vi "Main Engine Send Hardware Info.vi"(5 "Q Cluster":T6, 6 "Hardware Info":T1[](array[typedef]) {"Is Present?" items=["Initializing"=-2, "Unknown"=-1, "Not Present"=0, "Present"=1]}, 7 "DAQ Device Info":T8[](array[typedef]), 8 "error in":errorcluster, 9 "Ethernet IP Address":string[](array[string]), 10 "Serial Device Info":T7[](array[typedef])) -> (0 "error out":errorcluster)   [LabVIEW 2021]
doc: "All Rights Reserved © 2023 SyncSols"
uses:
  Controls/Main Engine DAQ Device Info.ctl
  Controls/Main Engine Serial Card Details.ctl
  Controls/Main Engine Q Cluster.ctl
  Controls/RT HW Info.ctl
  Controls/Main Engine Serial Info JSON Data.ctl
  Controls/Main Engine DAQ Harware Info JSON Data.ctl
  Controls/Main Engine Ehernet IP Address JSON Data.ctl
  Controls/Main Engine Hardware Info Data Cluster.ctl
  Host-Control's/TCP Tx-Rx cluster.ctl
  <vilib>/addons/_JKI.lib/Serialization/JSON/JKI JSON Serialization.lvlib
panel:
  in  "output cluster":T2
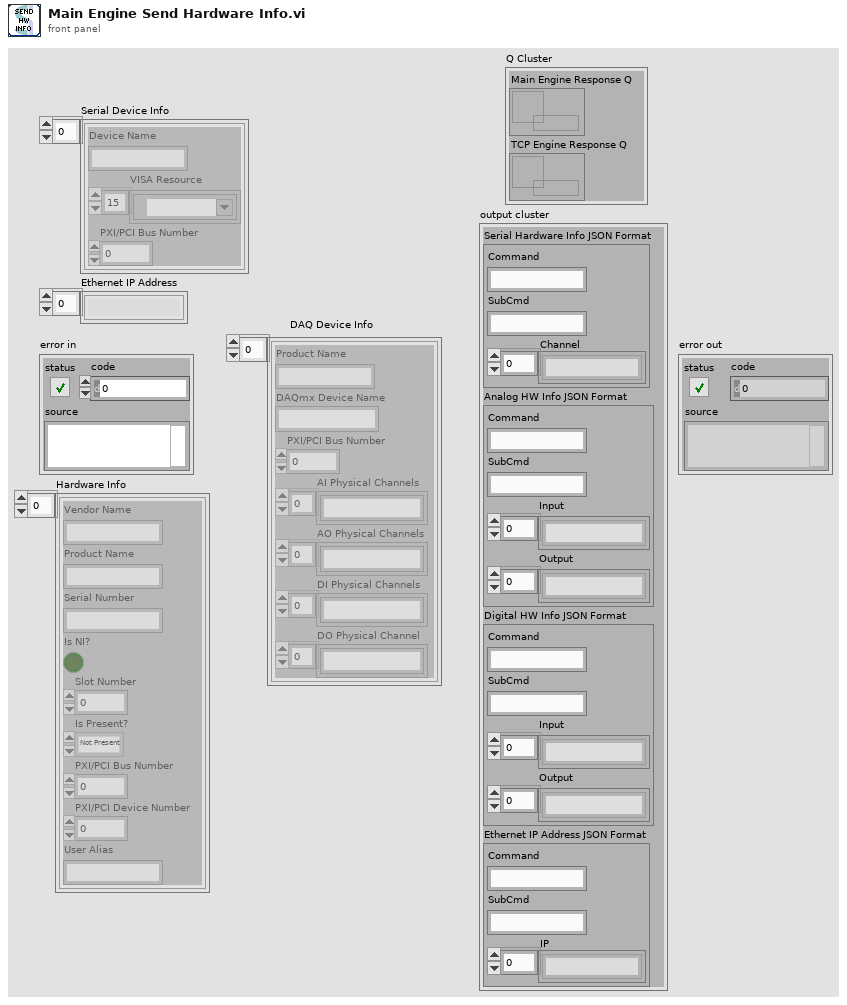
[diagram p1: front panel]
types:
  T1 = typedef "Main Engine Hardware Info Data Cluster.ctl" = cluster{"Vendor Name":string, "Product Name":string, "Serial Number":string, "Is NI?":bool, "Slot Number":i32, "Is Present?":i32, "PXI/PCI Bus Number":u32, "PXI/PCI Device Number":u32, "User Alias":string}
  T2 = typedef "RT HW Info.ctl" = cluster{"Serial Hardware Info JSON Format":T3, "Analog HW Info JSON Format":T4, "Digital HW Info JSON Format":T4, "Ethernet IP Address JSON Format":T5}
  T3 = typedef "Main Engine Serial Info JSON Data.ctl" = cluster{"Command":string, "SubCmd":string, "Channel":string[]}
  T4 = typedef "Main Engine DAQ Harware Info JSON Data.ctl" = cluster{"Command":string, "SubCmd":string, "Input":string[], "Output":string[]}
  T5 = typedef "Main Engine Ehernet IP Address JSON Data.ctl" = cluster{"Command":string, "SubCmd":string, "IP":string[]}
  T6 = typedef "Main Engine Q Cluster.ctl" = cluster{"Main Engine Response Q":refnum<queue>, "TCP Engine Response Q":refnum<queue>}
  T7 = typedef "Main Engine Serial Card Details.ctl" = cluster{"Device Name":string, "VISA Resource":refnum<visa-resource-name>[], "PXI/PCI Bus Number":u32}
  T8 = typedef "Main Engine DAQ Device Info.ctl" = cluster{"Product Name":string, "DAQmx Device Name":string, "PXI/PCI Bus Number":u32, "AI Physical Channels":string[], "AO Physical Channels":string[], "DI Physical Channels":string[], "DO Physical Channel":string[]}
  T9 = typedef "TCP Tx-Rx cluster.ctl" = cluster{"Interface":string, "Command":string, "SubCmd":string, "Data":variant}
  T10 = cluster{"DAQ Device Info":T8[], "Ethernet IP Address":string[]}
  T11 = cluster{"Serial Hardware Info JSON Format":T3, "Analog HW Info JSON Format":T4, "Digital HW Info JSON Format":T4, "Ethernet IP Address JSON Format":T5}
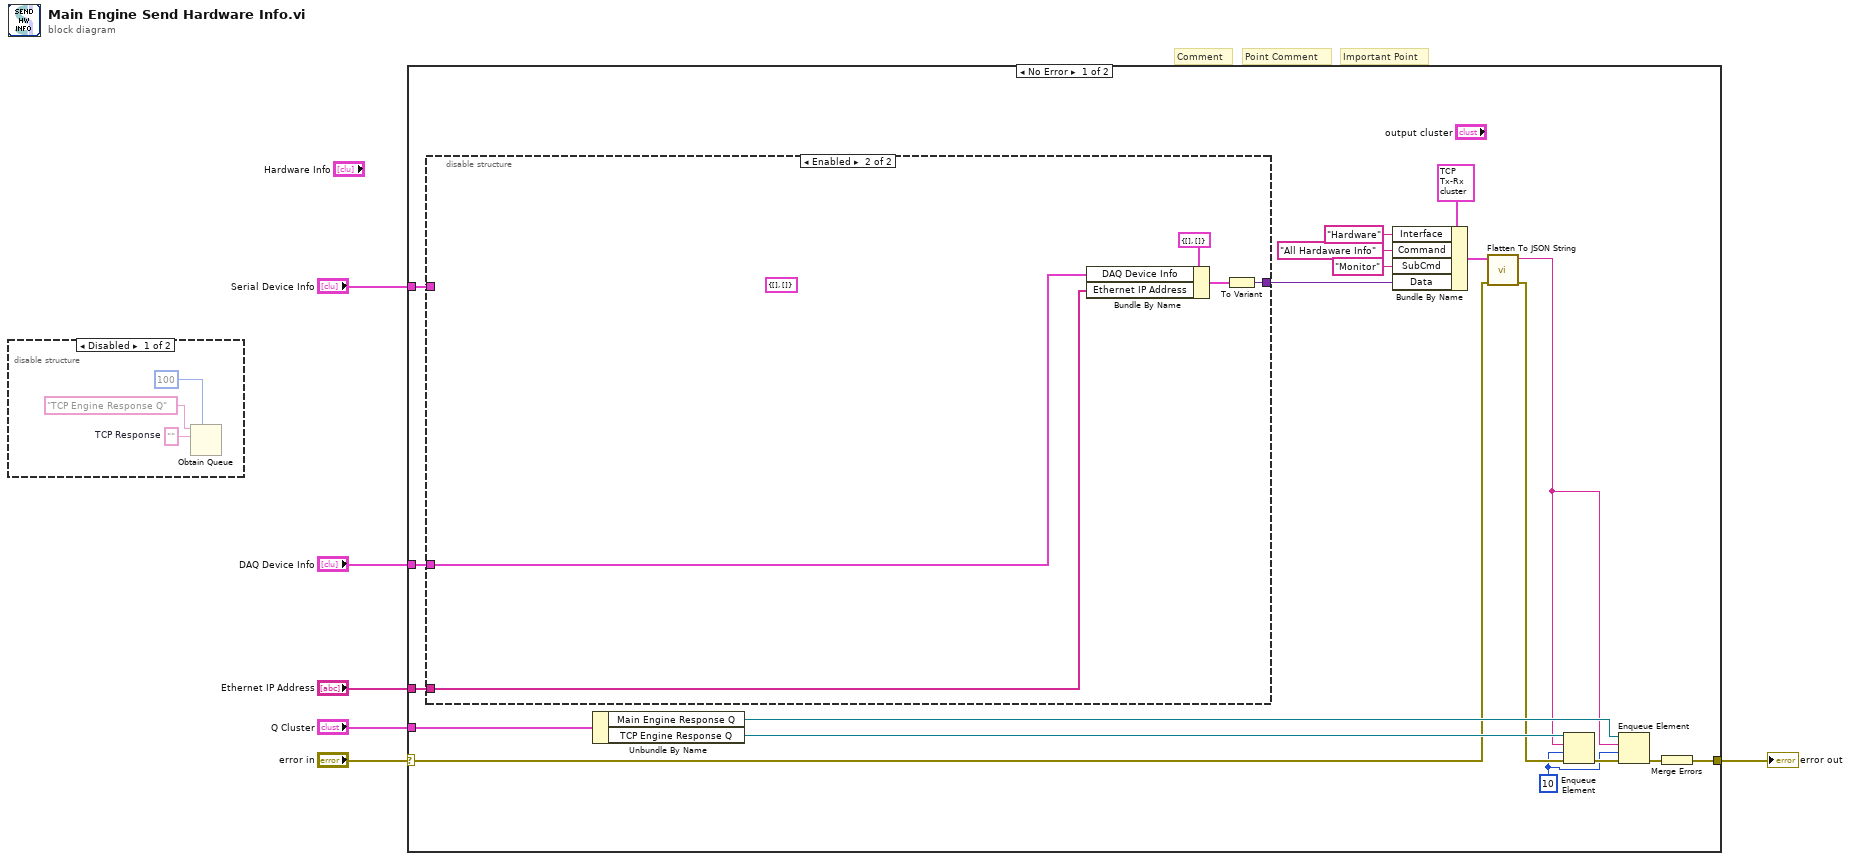
[diagram p0: block diagram]
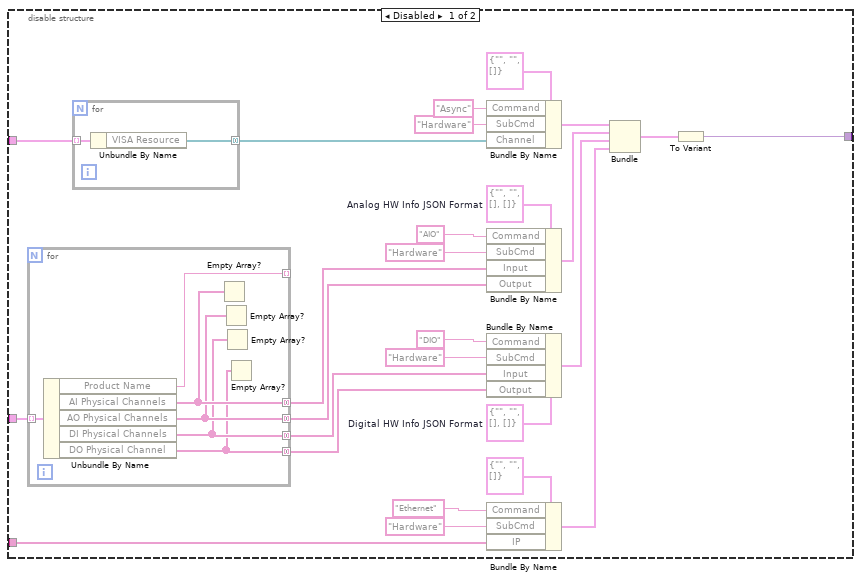
[diagram p3: hidden frame]
diagram:
  # "Important Point"
  # "Point Comment"
  # "Comment"
  n1 = disable-structure shown="Disabled" {
    frame Disabled {
      w9 = ""  # TCP Response
      n2 = Obtain Queue(max queue size (-1, unlimited)=100, name (unnamed)="TCP Engine Response Q", element data type=w9) -> ()  [unwired: 2 in, 3 out]
    }
    frame Enabled {
    }
  }
  n3 = case shown="No Error" "error in" {
    selector: "error in" -> [w13 w68]
    tunnel: [w25 w68] -> w6
    tunnel: "DAQ Device Info" -> [w28 _]
    tunnel: "Serial Device Info" -> [w27 _]
    tunnel: "Ethernet IP Address" -> [w23 _]
    tunnel: "Q Cluster" -> [w22 _]
    frame No Error {
      w10 = 10 ("timeout in ms (-1)")
      n4 = disable-structure shown="Enabled" {
        disable-tunnel: w28 -> [w54 w63]
        disable-tunnel: w27 -> [w48 _]
        disable-tunnel: w23 -> [w36 w66]
        disable-tunnel: [w29 w67] -> w16
        frame Disabled {
          w51 = T4 {"Command"="", "SubCmd"="", "Input"=[], "Output"=[]}  # Digital HW Info JSON Format
          w34 = T4 {"Command"="", "SubCmd"="", "Input"=[], "Output"=[]}  # Analog HW Info JSON Format
          n5 = for {
            tunnel: w54 -> [w57] mode=indexing
            tunnel: [w61] -> w43 mode=concatenating
            tunnel: [w60] -> w42 mode=concatenating
            tunnel: [w59] -> w41 mode=concatenating
            tunnel: [w58] -> w40 mode=concatenating
            tunnel: [w62] -> _ mode=indexing
            n6 = Unbundle By Name(w57) -> ("Product Name"=w62:string, "AI Physical Channels"=w61:string[], "AO Physical Channels"=w60:string[], "DI Physical Channels"=w59:string[], "DO Physical Channel"=w58:string[])
            n7 = Empty Array?(array=w61) -> ()  [unwired: 1 out]
            n8 = Empty Array?(array=w60) -> ()  [unwired: 1 out]
            n9 = Empty Array?(array=w59) -> ()  [unwired: 1 out]
            n10 = Empty Array?(array=w58) -> ()  [unwired: 1 out]
          }
          n11 = for {
            tunnel: w48 -> [w56] mode=indexing
            tunnel: [w55] -> w44 mode=concatenating
            n12 = Unbundle By Name(w56) -> ("VISA Resource"=w55:refnum<visa-resource-name>[])
          }
          n13 = Bundle By Name(cluster=T3 {"Command"="", "SubCmd"="", "Channel"=[]} ("Serial Hardware Info JSON Format"), "Command"="Async", "SubCmd"="Hardware" ("Sub Command"), "Channel"=w44) -> (w35:T3)
          n14 = Bundle By Name(cluster=w34, "Command"="AIO", "SubCmd"="Hardware" ("Sub Command"), "Input"=w43, "Output"=w42) -> (w31:T4)
          n15 = Bundle By Name(cluster=w51, "Command"="DIO", "SubCmd"="Hardware" ("Sub Command"), "Input"=w41, "Output"=w40) -> (w33:T4)
          n16 = Bundle By Name(cluster=T5 {"Command"="", "SubCmd"="", "IP"=[]} ("Ethernet IP Address JSON Format"), "Command"="Ethernet", "SubCmd"="Hardware" ("Sub Command"), "IP"=w36) -> (w32:T5)
          n17 = Bundle("Serial Hardware Info JSON Format"=w35, "Analog HW Info JSON Format"=w31, "Digital HW Info JSON Format"=w33, "Ethernet IP Address JSON Format"=w32) -> (w30:T11)  [unwired: 1 in]
          n18 = To Variant(anything=w30) -> (Variant=w29:variant)
        }
        frame Enabled {
          (unwired) T10 {"DAQ Device Info"=[], "Ethernet IP Address"=[]} ("output cluster")
          n19 = Bundle By Name(cluster=T10 {"DAQ Device Info"=[], "Ethernet IP Address"=[]} ("output cluster"), "DAQ Device Info"=w63, "Ethernet IP Address"=w66) -> (w65:T10)
          n20 = To Variant(anything=w65) -> (Variant=w67:variant)
        }
      }
      n21 = Unbundle By Name(w22) -> ("Main Engine Response Q"=w21:refnum<queue>, "TCP Engine Response Q"=w20:refnum<queue>)
      n22 = Bundle By Name(cluster=T9 {"Interface"="CPU", "Command"="CPU Info", "SubCmd"="Monitor", "Data"=variant} ("TCP Tx-Rx Cluster"), "Interface"="Hardware", "Command"="All Hardaware Info", "SubCmd"="Monitor" ("Interface Data.SubCmd"), "Data"=w16) -> (w15:T9)
      n23 = call <vilib>:"Flatten To JSON String.vi"("error in"=w13, "Variant"=w15) -> ("error out"=w12:errorcluster, "JSON String"=w11:string)  [unwired: 8 in]
      n24 = Enqueue Element(queue=w20, element=w11, timeout in ms (-1)=w10, error in (no error)=w12) -> (error out=w24:errorcluster)  [unwired: 2 out]
      n25 = Enqueue Element(queue=w21, element=w11, timeout in ms (-1)=w10, error in (no error)=w24) -> (error out=w26:errorcluster)  [unwired: 2 out]
      n26 = Merge Errors(w26) -> (w25:errorcluster)
    }
    frame Error {
    }
  }
  "error out" <- w6
